vi "RT Main.vi"() -> ()   [LabVIEW 2019]
doc: "The NI ELVIS III Custom FPGA Project template acquires button data from the onboard button and displays the button value on a Boolean indicator."
uses:
  <vilib>/rvi/interface/nirviReadWriteControl/nirviReadWriteControl.xnode
  <vilib>/myRIO/Instrument Drivers/Utilities/Utilities.lvlib
  <vilib>/rvi/interface/nirviCloseFPGA/nirviCloseFPGA.xnode
  <vilib>/rvi/interface/nirviOpenFPGA/nirviOpenFPGA.xnode
  NiFpgaLv.dll
  <vilib>/Utility/error.llb/Error Cluster From Error Code.vi
  <vilib>/rvi/interface/Simulation/niFpgaSimulationCallBeginRW.vi
  <vilib>/rvi/errors/niLvFpgaAdjustHostInterfaceError.vi
  <vilib>/FPGAPlugInAG/Dynamic/niLvFpga_Close_Dynamic.vi
  FPGA Main Default.vi
panel:
  out "Button Value":bool
  out "error out":errorcluster
  in  "Stop":bool
  # "ELVIS III Control IO"
  # "模拟控制IO"
  # "Overview: The NI ELVIS III Custom FPGA Project template acquires button data from the onboard button and displays the button value on a Boolean indicator.\nRequirements: \n1. LabVIEW FPGA Module.\n2. Xilinx Compilation Tools.\nInstructions:\n1. Check the NI ELVIS III target IP address in the project and make sure the target IP address is correct. \n2. Run this VI.\n3. Press the button on the NI ELVIS III device."
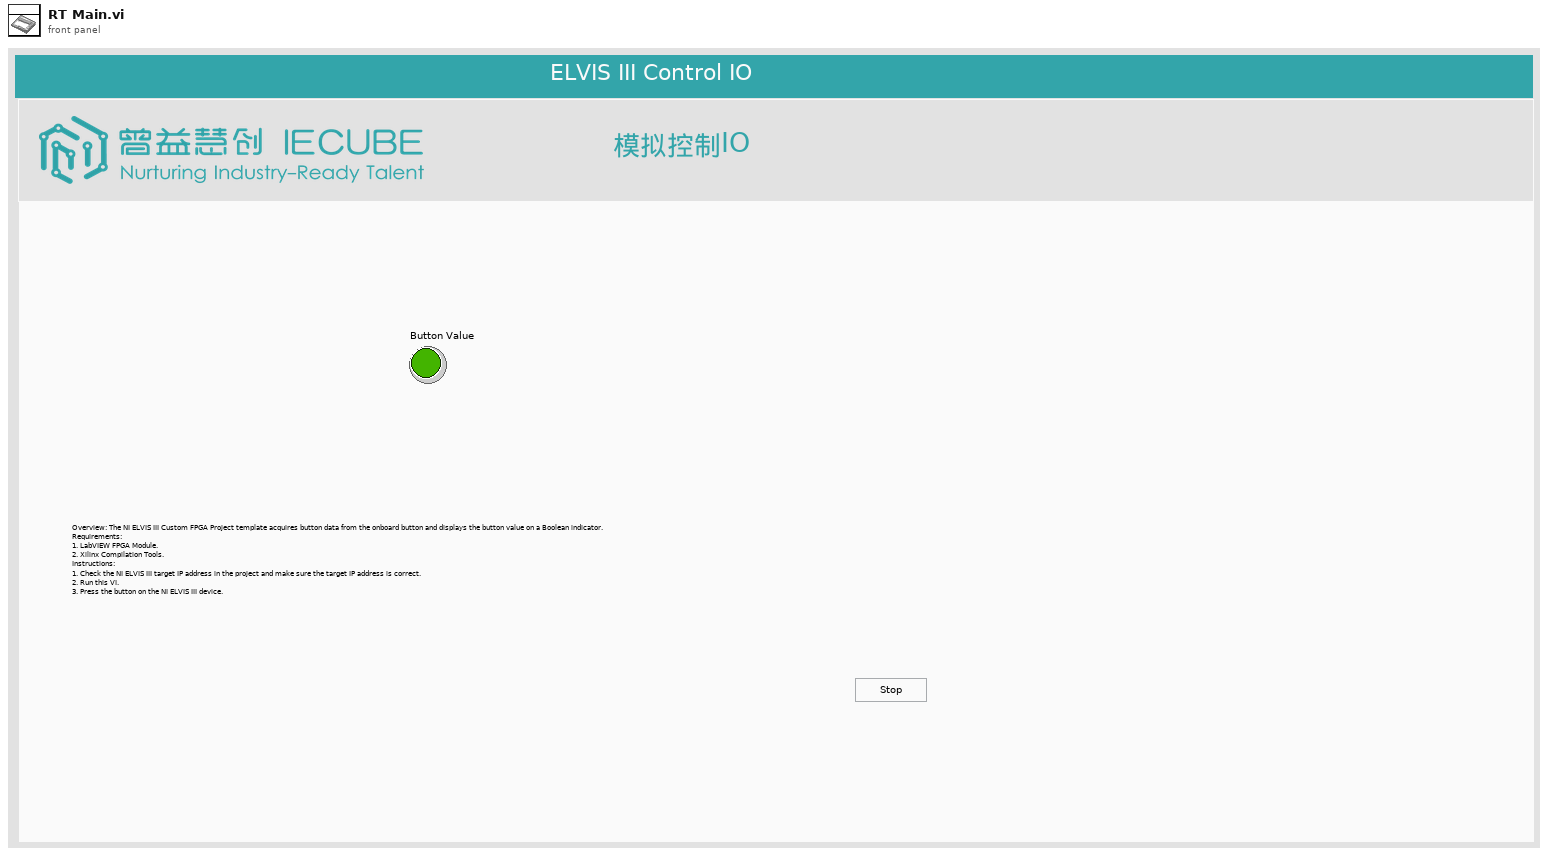
[diagram p1: front panel]
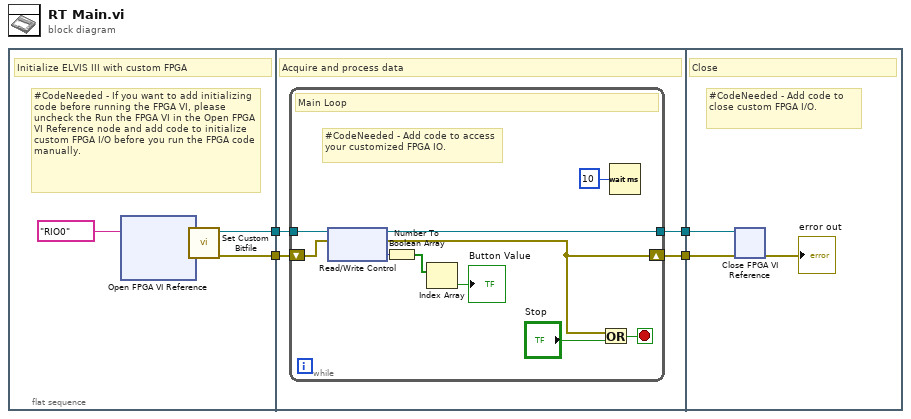
[diagram p0: block diagram]
diagram:
  n1 = flat-sequence {
    tunnel: [w6] -> w4
    tunnel: [w7] -> w3
    tunnel: w4 -> [w13]
    tunnel: w3 -> [w12]
    tunnel: [w11] -> w2
    tunnel: [w10] -> w1
    tunnel: w2 -> [w26]
    tunnel: w1 -> [w25]
    frame #0 {
      # "#CodeNeeded - If you want to add initializing code before running the FPGA VI, please uncheck the Run the FPGA VI in the Open FPGA VI Reference node and add code to initialize custom FPGA I/O before you run the FPGA code manually."
      # "Initialize ELVIS III with custom FPGA"
      n2 = xnode "Open FPGA VI Reference"("资源名称"=tag "RIO0" ("resource name")) -> ("FPGA VI引用输出"=w8:refnum<k20>, "错误输出"=w9:errorcluster)  [unwired: 1 in]
      n3 = call <vilib>:"Set Custom Bitfile.vi"("error in (no error)"=w9, "Custom FPGA Reference In"=w8) -> ("error out"=w6:errorcluster, "Custom FPGA Reference Out"=w7:refnum<k20>)  [unwired: 8 in]
    }
    frame #1 {
      # "Acquire and process data"
      n4 = while {
        tunnel: w12 -> [w21]
        tunnel: [w19] -> w11
        shift-right: [w17] -> w10
        shift-left: w13 -> [w18]
        stop <- w22 stop-if-true
        # "#CodeNeeded - Add code to access your customized FPGA IO."
        # "Main Loop"
        n5 = xnode "Read/Write Control"("FPGA VI引用输入"=w21, "错误输入"=w18) -> ("FPGA VI引用输出"=w19:refnum<k20>, "错误输出"=w17:errorcluster, "DI.BTN"=w16:u8)
        n6 = Number To Boolean Array(number=w16) -> (Boolean array=w15:bool[])
        n7 = Index Array(array=w15) -> (element=→"Button Value":bool)  [unwired: 1 in]
        n8 = Or(x=w17, y="Stop") -> (x .or. y?=w22:bool)
        n9 = Wait (ms)(milliseconds to wait=u32 10) -> ()  [unwired: 1 out]
      }
    }
    frame #2 {
      # "#CodeNeeded - Add code to close custom FPGA I/O."
      # "Close"
      n10 = xnode "Close FPGA VI Reference"("FPGA VI引用输入"=w26, "错误输入"=w25) -> ("错误输出"=→"error out":errorcluster)
    }
  }
